vi "Log to Host.vi"(8 "error in":errorcluster, 10 "Detail":string, 11 "MSS Target Actor in":refnum<class "MSS Target Actor.lvclass">) -> (0 "error out":errorcluster, 3 "MSS Target Actor out":refnum<class "MSS Target Actor.lvclass">)   [LabVIEW 2023, in "MSS Target Actor.lvlib" / "MSS Target Actor.lvclass"]
uses:
  MSS Target Actor.lvclass
  Study/Study Actor/IStudy Actor Messages/Log Target Msg/Log Target Msg.lvclass/Log Target Msg.ctl
  <vilib>/ActorFramework/Message Enqueuer/Message Enqueuer.lvclass/Message Enqueuer.ctl
  <vilib>/ActorFramework/Message Enqueuer/Enqueue.vi
  Study/Study Actor/IStudy Actor Messages/Log Target Msg/Log Target Msg.lvclass
  <vilib>/Utility/LVClass/Get LV Class Name.vi
  <resource>/AFDebug/Generate Trace for Message.vi
  <vilib>/ActorFramework/Message Priority Queue/Priority Enqueue.vi
  MSS Target Actor.lvclass/MSS Target Actor.ctl
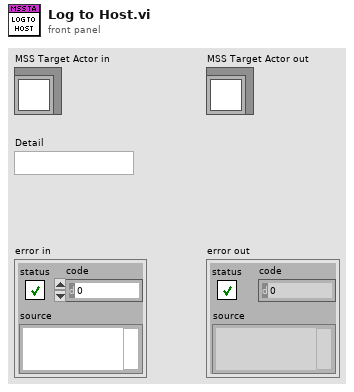
[diagram p1: front panel]
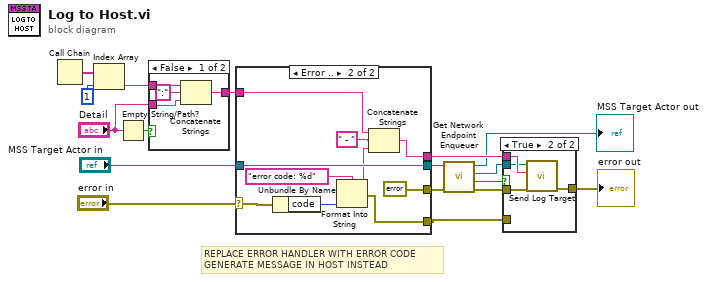
[diagram p0: block diagram]
diagram:
  # "REPLACE ERROR HANDLER WITH ERROR CODE\nGENERATE MESSAGE IN HOST INSTEAD"
  n1 = Call Chain() -> (call chain=w6:string[])
  n2 = Index Array(array=w6, index=1) -> (element=w4:string)
  n3 = Empty String/Path?(string/path="Detail") -> (empty?=w3:bool)
  n4 = case shown="False" w3 {
    tunnel: w4 -> [w21 w22]
    tunnel: "Detail" -> [w19 _]
    tunnel: [w18 w22] -> w1
    frame False {
      n5 = Concatenate Strings(w21, ":" ("string"), w19) -> (w18:string)
    }
    frame True {
    }
  }
  n6 = case shown="Error .." "error in" {
    selector: "error in" -> [w25 w29]
    tunnel: "MSS Target Actor in" -> [w24 w35]
    tunnel: [w24 w35] -> w12
    tunnel: [w23 w33] -> w11
    tunnel: [w25 errorcluster {"status"=FALSE, "code"=0, "source"=""} ("error in (no error)")] -> w9
    tunnel: [_ w26] -> w8
    tunnel: w1 -> [w23 w31]
    frame No Error {
    }
    frame Error {
      n7 = Unbundle By Name(w29) -> ("code"=w30:i32)
      n8 = Format Into String(format string="error code: %d", w30) -> (resulting string=w27:string, error out=w26:errorcluster)  [unwired: 2 in]
      n9 = Concatenate Strings(w31, " - " ("string"), w27) -> (w33:string)
    }
  }
  n10 = call "Get Network Endpoint Enqueuer.vi"("error in"=w9, "MSS Target Actor in"=w12) -> ("error out"=w16:errorcluster, "Connected?"=w15:bool, "Enqueuer"=w10:refnum<class "Message Enqueuer.lvclass">, "MSS Target Actor out"=→"MSS Target Actor out":refnum<class "MSS Target Actor.lvclass">)  [unwired: 6 in]
  n11 = case shown="True" w15 {
    tunnel: w16 -> [_ w37]
    tunnel: w11 -> [_ w40]
    tunnel: [w36 w39] -> w17
    tunnel: w10 -> [_ w38]
    tunnel: w8 -> [w36 _]
    frame False {
    }
    frame True {
      n12 = call "Send Log Target.vi"("error in (no error)"=w37, "Entry"=w40, "Message Enqueuer"=w38) -> ("error out"=w39:errorcluster)  [unwired: 7 in, 1 out]
    }
  }
  "error out" <- w17
